vi "ADAM6052.vi"() -> ()   [LabVIEW 2014]
uses:
  <vilib>/NI Modbus.llb/MB Modbus Command.ctl
  <vilib>/NI Modbus.llb/MB Ethernet Master Query Write Multiple Coils (poly).vi
  <vilib>/NI Modbus.llb/MB Ethernet Master Query Read Coils (poly).vi
panel:
  out "Coils":bool[](array[boolean])
  out "TCP Network Connection Refnum":refnum<k5>
  out "error out":errorcluster
  in  "error in (no error)":errorcluster
  in  "remote port":u16=502
  in  "address":string="192.168.100.1"
  in  "Discrete":bool[](array[boolean])
  in  "stop":bool
  in  "Modbus Command":T1={"Function Code"=15, "Starting Address"=17, "Quantity"=4, "Data"=[], "Discrete"=[]} {"Function Code" items=["Read Coils"=1, "Read Discrete Inputs"=2, "Read Holding Registers"=3, "Read Input Registers"=4, "Write Single Coil"=5, "Write Single Register"=6, "Read Exception Status"=7, "Write Multiple Coils"=15, "Write Multiple Registers"=16]}
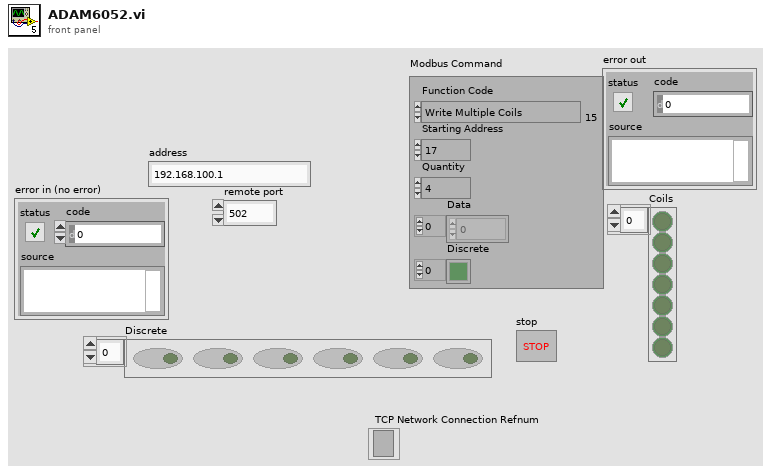
[diagram p1: front panel]
types:
  T1 = typedef "MB Modbus Command.ctl" = cluster{"Function Code":u8, "Starting Address":u16, "Quantity":u16, "Data":u16[], "Discrete":bool[]}
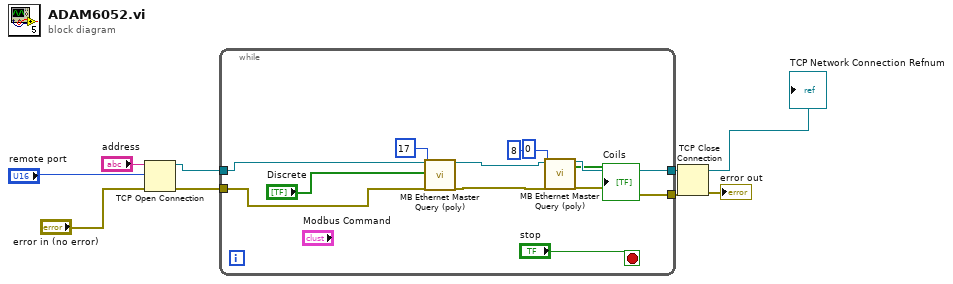
[diagram p0: block diagram]
diagram:
  n1 = TCP Open Connection(address="address", remote port or service name="remote port", error in (no error)="error in (no error)") -> (connection ID=w8:refnum<k5>, error out=w5:errorcluster)  [unwired: 2 in]
  n2 = while {
    tunnel: [w11] -> w1
    tunnel: w8 -> [w19]
    tunnel: w5 -> [w16]
    tunnel: [w12] -> w4
    stop <- "stop" stop-if-true
    n3 = call-poly <vilib>:"MB Ethernet Master Query (poly).vi"("TCP Connection Refnum in"=w19, "Starting Address"=u16 17, "Coils"="Discrete", "error in"=w16) -> ("TCP Connection Refnum (dup)"=w10:refnum<k5>, "error out"=w13:errorcluster)  [unwired: 13 in, 1 out]
    n4 = call-poly <vilib>:"MB Ethernet Master Query (poly).vi"("TCP Connection Refnum in"=w10, "Starting Address"=u16 0, "Quantity"=u16 8, "error in"=w13) -> ("TCP Connection Refnum (dup)"=w11:refnum<k5>, "Coils"=→"Coils":bool[], "error out"=w12:errorcluster)  [unwired: 12 in, 1 out]
  }
  "TCP Network Connection Refnum" <- w1
  n5 = TCP Close Connection(connection ID=w1, error in (no error)=w4) -> (error out=→"error out":errorcluster)  [unwired: 1 in, 1 out]
